vi "X-Design Filter.vi"(6 "order":i32=2, 8 "error in (no error)":errorcluster, 10 "Filter settings":cluster{"Highpass (Hz)":dbl, "Lowpass (Hz)":dbl}={"Highpass (Hz)"=300.0, "Lowpass (Hz)"=3000.0}, 11 "sampling freq: fs":dbl=1.0 format="%0.2f") -> (0 "error out":errorcluster, 3 "IIR Filters":T1(array[cluster]))   [LabVIEW 2020]
uses:
  <vilib>/Analysis/3filter.llb/Filter Passband Type.ctl
  <vilib>/Analysis/NI_AALBase.lvlib
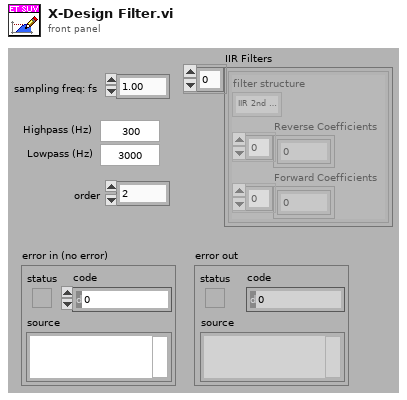
[diagram p1: front panel]
types:
  T1 = cluster{"filter structure":enum32{"IIR 2nd Order", "IIR 4th Order"}, "Reverse Coefficients":dbl[], "Forward Coefficients":dbl[]}[]
  T2 = typedef "NI_AALBase.lvlib/Filter Passband Type.ctl" = enum32{"Lowpass", "Highpass", "Bandpass", "Bandstop"}
  T3 = cluster{"filter structure":enum32{"IIR 2nd Order", "IIR 4th Order"}, "Reverse Coefficients":dbl[], "Forward Coefficients":dbl[]}
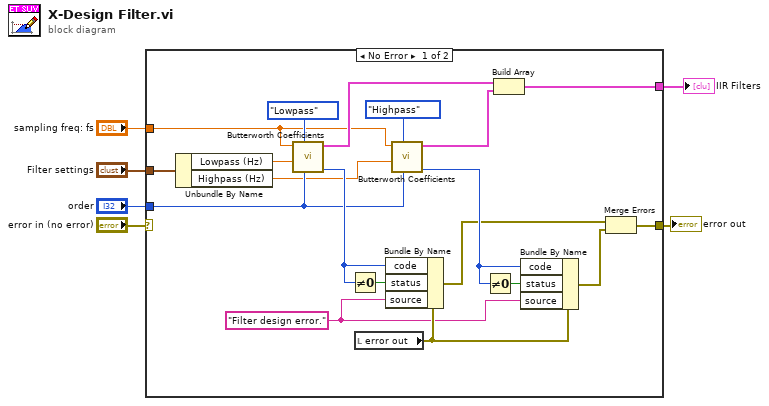
[diagram p0: block diagram]
diagram:
  n1 = case shown="No Error" "error in (no error)" {
    selector: "error in (no error)" -> [_ w26]
    tunnel: "order" -> [w20 _]
    tunnel: "sampling freq: fs" -> [w19 _]
    tunnel: [w14 w26] -> w4
    tunnel: [w10 _] -> w3
    tunnel: "Filter settings" -> [w9 _]
    frame No Error {
      w15 = "Filter design error." ("source")
      n2 = Unbundle By Name(w9) -> ("Lowpass (Hz)"=w8:dbl, "Highpass (Hz)"=w7:dbl)
      n3 = call <vilib>:"Butterworth Coefficients.vi"("order"=w20, "filter type"=Filter_Passband_Type."Lowpass", "low cutoff freq: fl"=w8, "sampling freq: fs"=w19) -> ("error"=w23:i32, "IIR Filter Cluster"=w25:T3)  [unwired: 6 in]
      n4 = Not Equal To 0?(x=w23) -> (x != 0?=w24:bool)
      n5 = local read "error out"() -> (w16:errorcluster)
      n6 = Bundle By Name(cluster=w16, "code"=w23, "status"=w24, "source"=w15) -> (w12:errorcluster)
      n7 = call <vilib>:"Butterworth Coefficients.vi"("order"=w20, "filter type"=Filter_Passband_Type."Highpass", "low cutoff freq: fl"=w7, "sampling freq: fs"=w19) -> ("error"=w17:i32, "IIR Filter Cluster"=w11:T3)  [unwired: 6 in]
      n8 = Not Equal To 0?(x=w17) -> (x != 0?=w18:bool)
      n9 = Build Array(w25, w11) -> (w10:T1)
      n10 = Bundle By Name(cluster=w16, "code"=w17, "status"=w18, "source"=w15) -> (w13:errorcluster)
      n11 = Merge Errors(w12, w13) -> (w14:errorcluster)
    }
    frame Error {
    }
  }
  "error out" <- w4
  "IIR Filters" <- w3
